vi "Skip to RPC Outputs.vi"(11 "String in":string) -> (1 "inputs":u8, 2 "Aborted":bool, 3 "String out":string)   [LabVIEW 2017]
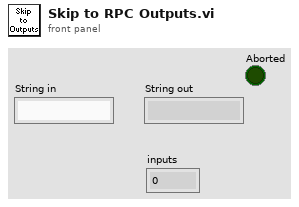
[diagram p1: front panel]
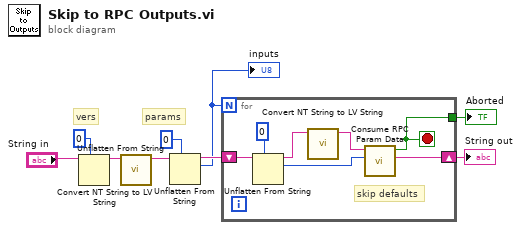
[diagram p0: block diagram]
diagram:
  # "params"
  # "vers"
  n1 = Unflatten From String(type=u8 0 ("bytes to read"), binary string="String in") -> (rest of the binary string=w4:string)  [unwired: 3 in, 2 out]
  n2 = call <vilib>:"Convert NT String to LV String.vi"("Buffer in"=w4) -> ("Remaining String"=w6:string)  [unwired: 8 in, 2 out]
  n3 = Unflatten From String(type=u8 0 ("bytes to read"), binary string=w6) -> (rest of the binary string=w8:string, value=w1:u8)  [unwired: 3 in, 1 out]
  "inputs" <- w1
  n4 = for {
    N: w1 -> [_]
    shift-right: [w13] -> w9
    shift-left: w8 -> [w15]
    tunnel: [w12] -> w2
    stop <- w12 stop-if-true
    # "skip defaults"
    n5 = Unflatten From String(type=u8 0 ("bytes to read"), binary string=w15) -> (rest of the binary string=w14:string, value=w11:u8)  [unwired: 3 in, 1 out]
    n6 = call <vilib>:"Convert NT String to LV String.vi"("Buffer in"=w14) -> ("Remaining String"=w10:string)  [unwired: 8 in, 2 out]
    n7 = call <vilib>:"Consume RPC Param Data.vi"("type"=w11, "RPC String in"=w10) -> ("string out"=w13:string, "Issue"=w12:bool)  [unwired: 6 in, 2 out]
  }
  "String out" <- w9
  "Aborted" <- w2
